vi "Colorbox to Hex.vi"(11 "Color Picker":u32) -> (0 "B":u8, 1 "G":u8, 2 "R":u8, 3 "HEx String":string)   [LabVIEW 2019, in "LSS.lvlib"]
uses:
  LSS.lvlib
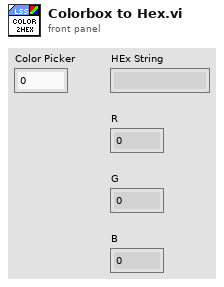
[diagram p1: front panel]
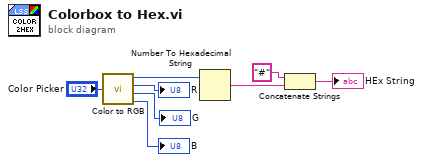
[diagram p0: block diagram]
diagram:
  n1 = call <vilib>:"Color to RGB.vi"("Color"="Color Picker") -> ("Resolved Color"=w6:u32, "R"=→"R":u8, "G"=→"G":u8, "B"=→"B":u8)
  n2 = Number To Hexadecimal String(2:w6) -> (0:w5:string)  [unwired: 1 in]
  n3 = Concatenate Strings("#" ("string"), w5) -> (→"HEx String":string)
